vi "um to ns.vi"(9 "# of path lengths (def.: 2)":i32=2, 10 "position (microns)":dbl[unit]) -> (2 "position (ns)":dbl[unit])   [LabVIEW 2009]
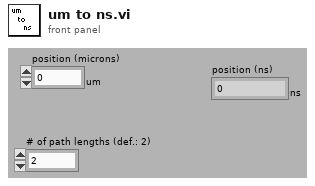
[diagram p1: front panel]
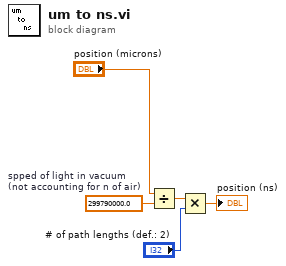
[diagram p0: block diagram]
diagram:
  w5 = dbl[unit] 299790000.0  # spped of light in vacuum (not accounting for n of air)
  n1 = Divide(x="position (microns)", y=w5) -> (x/y=w4:dbl[unit])
  n2 = Multiply(x=w4, y="# of path lengths (def.: 2)") -> (x*y=→"position (ns)":dbl[unit])
